vi "YKGS200_VoltageSweep.vi"() -> ()   [LabVIEW 2017]
doc: "This example shows how to configure the instrument's output voltage level, over current protection. The actual current level is returned as well as whether over current high or low protection (OCP) has been tripped."
uses:
  <vilib>/measure/NI_MABase.lvlib
panel:
  in  "Type":u16(ring) items=["Constant", "Triangle", "Sawtooth", "Sine", "Square"]
  in  "Output":cluster{"Amp (V)":dbl, "Freq (Hz)":dbl}={"Amp (V)"=0.1, "Freq (Hz)"=0.01}
  in  "Stop Output":bool
  out "OCP High Tripped?":bool
  out "OCP Low Tripped?":bool
  out "Actual Current Level (A)":dbl format="%.2p"
  in  "Current Limit (0.2 A)":dbl=0.2 min=0.001 max=0.2 format="%.3g"
  in  "VISA resource name":refnum<visa-resource-name>
  # "(c) 2010 Yokogawa Electric Corporation.  ALL RIGHTS RESERVED."
  # "Over Current Protection"
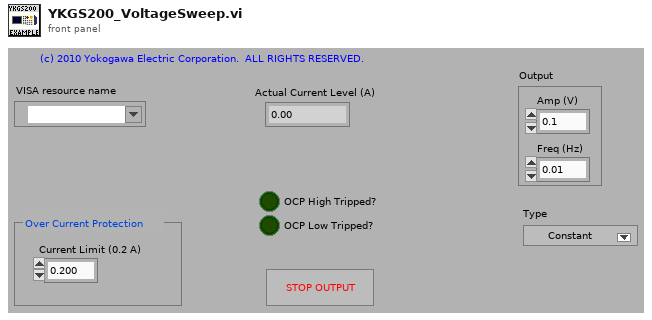
[diagram p1: front panel]
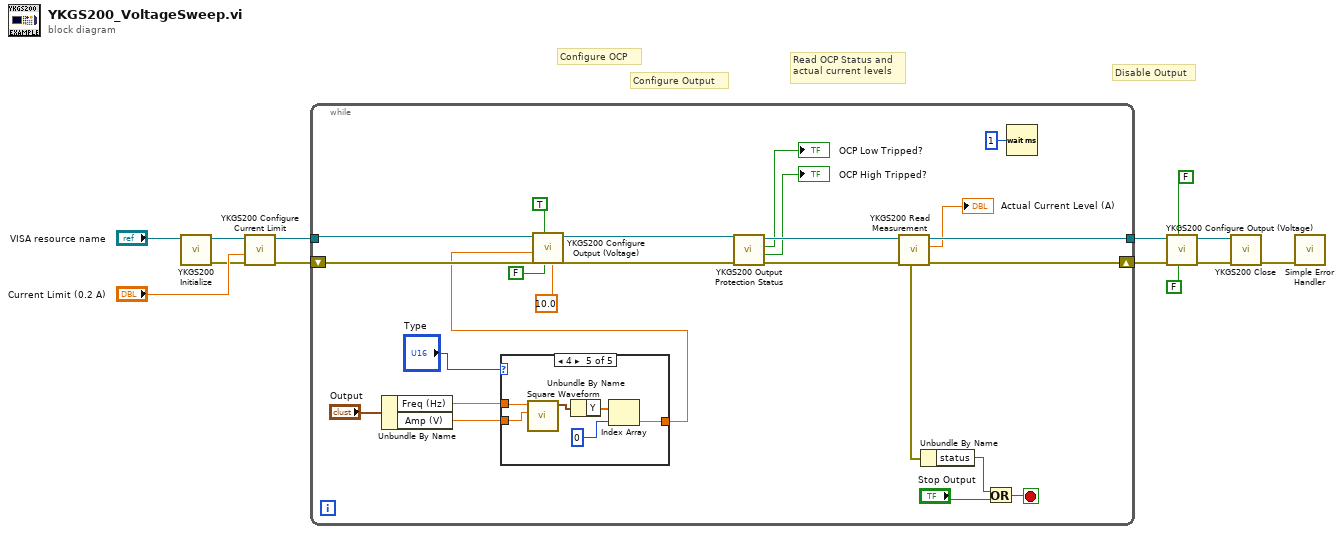
[diagram p0: block diagram]
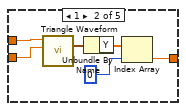
[diagram p3: hidden frame]
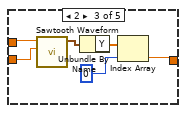
[diagram p4: hidden frame]
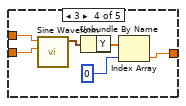
[diagram p5: hidden frame]
diagram:
  # "Disable Output"
  # "Read OCP Status and\nactual current levels"
  # "Configure Output"
  # "Configure OCP"
  n1 = call <instrlib>:"YKGS200 Initialize.vi"("VISA resource name"="VISA resource name") -> ("error out"=w4:errorcluster, "VISA resource name out"=w3:refnum<visa-resource-name>)  [unwired: 9 in]
  n2 = call <instrlib>:"YKGS200 Configure Current Limit.vi"("error in (no error)"=w4, "Current Limit (0.2 A)"="Current Limit (0.2 A)", "VISA resource name"=w3) -> ("error out"=w1:errorcluster, "VISA resource name out"=w2:refnum<visa-resource-name>)  [unwired: 7 in]
  n3 = while {
    tunnel: w2 -> [w25]
    tunnel: [w34] -> w12
    shift-right: [w27] -> w11
    shift-left: w1 -> [w35]
    stop <- w29 stop-if-true
    n4 = Unbundle By Name("Output") -> ("Freq (Hz)"=w18:dbl, "Amp (V)"=w17:dbl)
    n5 = case shown="4" "Type" {
      tunnel: w18 -> [_ w39 w46 w50 w56]
      tunnel: w17 -> [w36 w38 w45 w51 w57]
      tunnel: [w36 w37 w43 w49 w55] -> w15
      frame 0, Default {
      }
      frame 1 {
        n6 = call <vilib>:"Triangle Waveform.vi"("amplitude"=w38, "frequency"=w39) -> ("signal out"=w42:waveform(dbl))  [unwired: 8 in, 1 out]
        n7 = Unbundle By Name(w42) -> ("Y"=w41:dbl[])
        n8 = Index Array(array=w41, index=0) -> (element=w37:dbl)
      }
      frame 2 {
        n9 = call <vilib>:"Sawtooth Waveform.vi"("amplitude"=w45, "frequency"=w46) -> ("signal out"=w44:waveform(dbl))  [unwired: 8 in, 1 out]
        n10 = Unbundle By Name(w44) -> ("Y"=w48:dbl[])
        n11 = Index Array(array=w48, index=0) -> (element=w43:dbl)
      }
      frame 3 {
        n12 = call <vilib>:"Sine Waveform.vi"("amplitude"=w51, "frequency"=w50) -> ("signal out"=w52:waveform(dbl))  [unwired: 8 in, 1 out]
        n13 = Unbundle By Name(w52) -> ("Y"=w54:dbl[])
        n14 = Index Array(array=w54, index=0) -> (element=w49:dbl)
      }
      frame 4 {
        n15 = call <vilib>:"Square Waveform.vi"("amplitude"=w57, "frequency"=w56) -> ("signal out"=w58:waveform(dbl))  [unwired: 8 in, 1 out]
        n16 = Unbundle By Name(w58) -> ("Y"=w60:dbl[])
        n17 = Index Array(array=w60, index=0) -> (element=w55:dbl)
      }
    }
    n18 = call <instrlib>:"YKGS200 Configure Output (Voltage).vi"("Voltage Range (.30 V)"=10.0, "Enable Auto Range (T: Enable)"=FALSE, "Enable Output (T: Enable)"=TRUE, "Voltage Level (0.0 V)"=w15, "VISA resource name"=w25) -> ("VISA resource name out"=w24:refnum<visa-resource-name>)  [unwired: 5 in, 1 out]
    n19 = call <instrlib>:"YKGS200 Output Protection Status.vi"("error in (no error)"=w35, "VISA resource name"=w24) -> ("error out"=w32:errorcluster, "High Limiting?"=→"OCP High Tripped?":bool, "Low Limiting?"=→"OCP Low Tripped?":bool, "VISA resource name out"=w33:refnum<visa-resource-name>)  [unwired: 6 in]
    n20 = call <instrlib>:"YKGS200 Read Measurement.vi"("error in (no error)"=w32, "VISA resource name"=w33) -> ("error out"=w27:errorcluster, "Actual Level"=→"Actual Current Level (A)":dbl, "VISA resource name out"=w34:refnum<visa-resource-name>)  [unwired: 7 in]
    n21 = Unbundle By Name(w27) -> ("status"=w26:bool)
    n22 = Or(x=w26, y="Stop Output") -> (x .or. y?=w29:bool)
    n23 = Wait (ms)(milliseconds to wait=u32 1) -> ()  [unwired: 1 out]
  }
  n24 = call <instrlib>:"YKGS200 Configure Output (Voltage).vi"("Enable Auto Range (T: Enable)"=FALSE, "Enable Output (T: Enable)"=FALSE, "error in (no error)"=w11, "VISA resource name"=w12) -> ("error out"=w9:errorcluster, "VISA resource name out"=w10:refnum<visa-resource-name>)  [unwired: 6 in]
  n25 = call <instrlib>:"YKGS200 Close.vi"("error in (no error)"=w9, "VISA resource name"=w10) -> ("error out"=w6:errorcluster)  [unwired: 9 in]
  n26 = call <vilib>:"Simple Error Handler.vi"("error in (no error)"=w6) -> ()  [unwired: 4 in, 5 out]
